vi "run_experiment_sCMOS_DAC_debug.vi"() -> ()   [LabVIEW 2015]
uses:
  <vilib>/addons/h5labview2/base/hid_t.ctl
  <vilib>/addons/h5labview2/base/H5Equery.vi
  <vilib>/addons/h5labview2/base/lib_path.vi
  <vilib>/DAQmx/write.llb/DAQmx Write (Digital Bool 1Line 1Point).vi
  <vilib>/addons/h5labview2/dataset/H5Dwrite.llb/H5Dwrite.xnode
  <vilib>/addons/h5labview2/dataset/H5D.lvlib
  <vilib>/addons/h5labview2/space/H5S.lvlib
  <vilib>/addons/h5labview2/file/H5F.lvlib
  <vilib>/DAQmx/read.llb/DAQmx Read (Analog 1D Wfm NChan NSamp).vi
  <vilib>/DAQmx/create/channels.llb/DAQmx Create Channel (DO-Digital Output).vi
  <vilib>/DAQmx/write.llb/DAQmx Write (Analog 1D DBL 1Chan NSamp).vi
panel:
  out "startrec err":errorcluster
  out "number of samples written per channel":u32
  out "error out 2":errorcluster
  out "temp .dcimg filepath":path
  out "Exposure":dbl
  out "V Width":i32
  out "H Width":i32
  out "Acquiring Frames":bool
  out "Frames Recorded":i32
  out "Display":T1(plugin-control)
  out "DAC Input":waveform(dbl)[](graph) caption="DAC Input Display"
  out "error out":errorcluster
  out "Current Stimulus Name":string
  out "Current Piezo Command":dynamicdata(graph)
  out "Current Stim Frames":i32
  out "Current Stim Duration":dbl
  out "Current Stimulus Save Path":path
  in  "Number Reps":dbl
  out "Experiment Path":path
  out "Timestamp":string
  out "Genotype":string
  out "Fly Name":string
  out "Experiment Name":string
  in  "Metadata Path":path
  out "Stimulus Files":path[](array[path])
  out "Num Stimuli":i32
  out "Protocol Name":string
  out "Protocol Rate":i32
  in  "Protocol Path":path
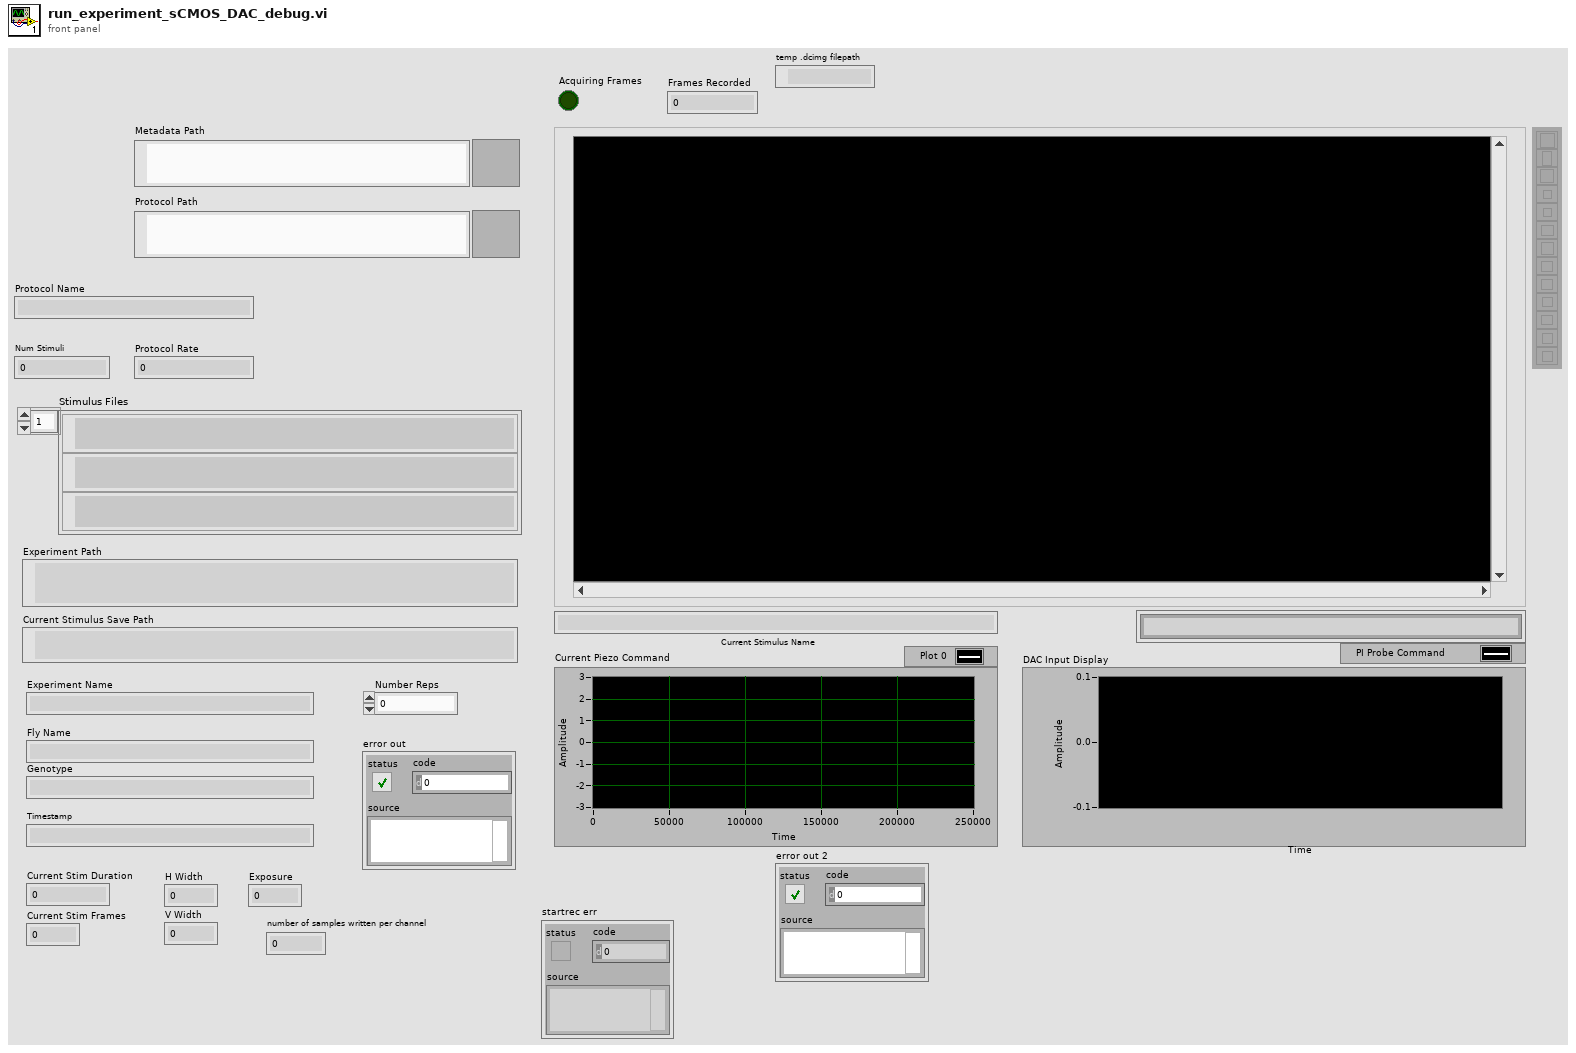
[diagram p1: front panel]
types:
  T1 = typedef "IMAQ Image.ctl" = refnum<image>
  T2 = cluster{"Value":i32, "Minimum":i32, "Maximum":i32, "Increment":i32}
  T3 = typedef "Image Type" = u32
  T4 = cluster{"height":u32, "width":u32, "datatype":u32}
  T5 = typedef "hid_t.ctl" = i32
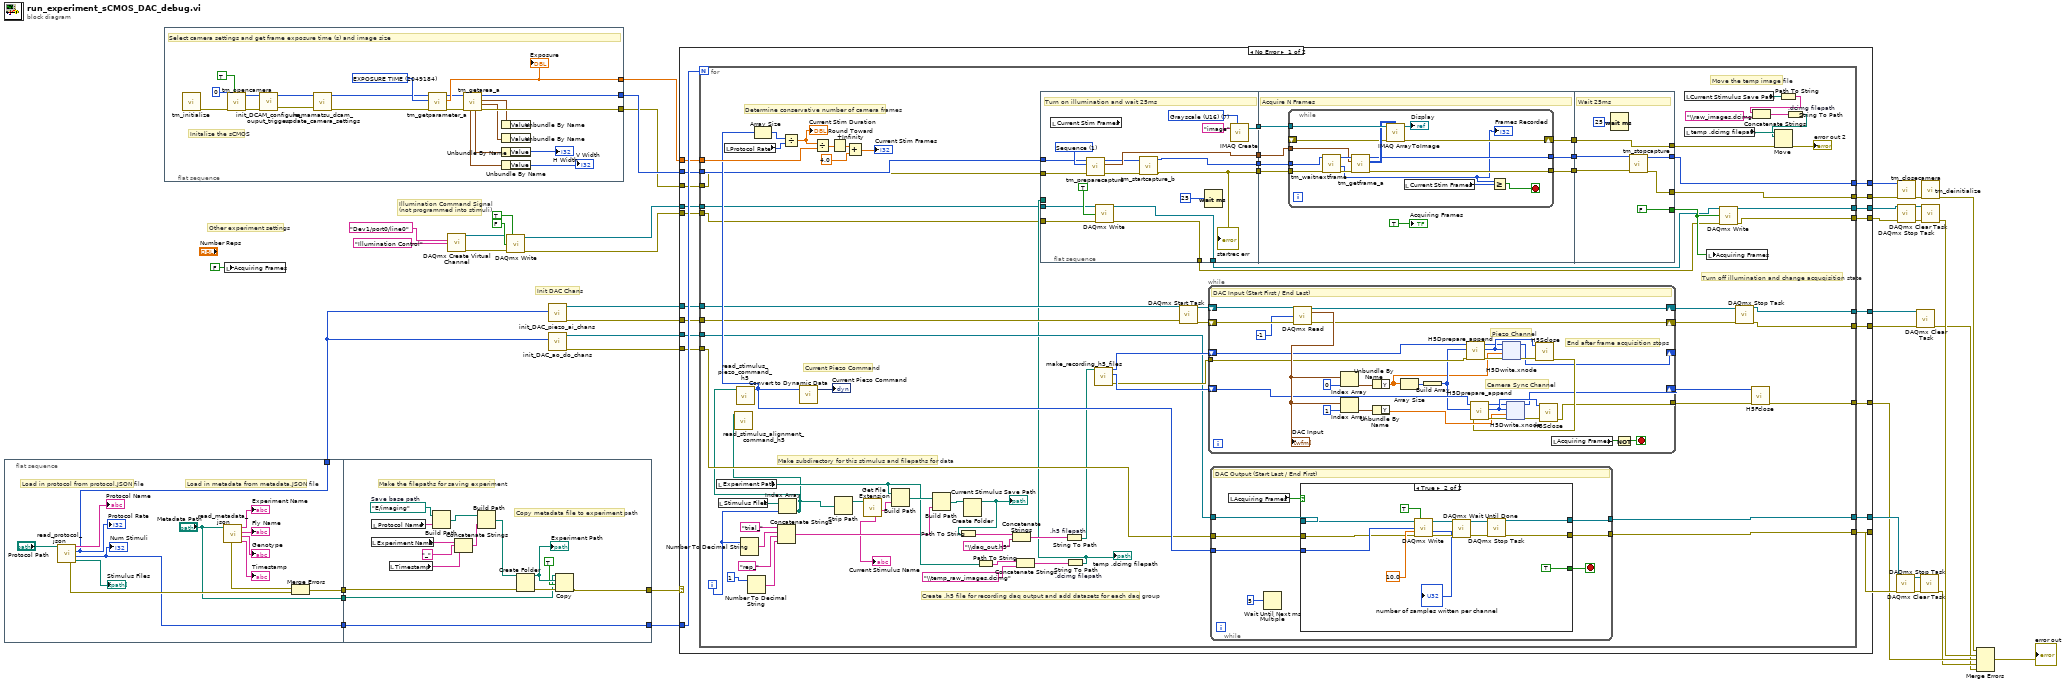
[diagram p0: block diagram]
diagram:
  # "Other experiment settings"
  # "Init DAC Chans"
  # "Illumination Command Signal \n(not programmed into stimuli)"
  n1 = flat-sequence {
    tunnel: [w44] -> w38
    tunnel: [w45] -> w10
    tunnel: ["Metadata Path"] -> w9
    tunnel: [w42] -> w8
    tunnel: [w69] -> w37
    tunnel: w10 -> [w57]
    tunnel: w9 -> [w56]
    tunnel: w8 -> [w69]
    tunnel: [w55] -> w7
    frame #0 {
      # "Load in metadata from metadata.JSON file"
      # "Load in protocol from protocol.JSON file"
      n2 = call "read_protocol_json.vi"("Path"="Protocol Path") -> ("stims"=→"Stimulus Files":path[], "n_stims"=w42:i32, "rate"=w44:i32, "protocol name"=→"Protocol Name":string, "error out"=w47:errorcluster)  [unwired: 6 in]
      "Protocol Rate" <- w44
      "Num Stimuli" <- w42
      n3 = call "read_metadata_json.vi"("Path"="Metadata Path") -> ("exp_time"=→"Timestamp":string, "genotype"=→"Genotype":string, "fly_name"=→"Fly Name":string, "exp_ name"=→"Experiment Name":string, "error out"=w46:errorcluster)  [unwired: 6 in]
      n4 = Merge Errors(w46, w47) -> (w45:errorcluster)
    }
    frame #1 {
      w64 = path "E:/imaging"  # Save base path
      # "Copy metadata file to experiment path"
      # "Make the filepaths for saving experiment"
      n5 = local read "Experiment Name"() -> (w61:string)
      n6 = local read "Protocol Name"() -> (w63:string)
      n7 = local read "Timestamp"() -> (w59:string)
      n8 = Build Path(base path=w64, name or relative path=w63) -> (appended path=w62:path)
      n9 = Concatenate Strings(w61, "_", w59) -> (w58:string)
      n10 = Build Path(base path=w62, name or relative path=w58) -> (appended path=w65:path)
      n11 = Create Folder(path (use dialog)=w65, error in=w57) -> (created path=w68:path, error out=w67:errorcluster)  [unwired: 1 in, 1 out]
      "Experiment Path" <- w68
      n12 = Copy(8:w67, 9:TRUE ("overwrite (F)"), 10:w68, 11:w56) -> (0:w55:errorcluster)  [unwired: 1 in, 2 out]
    }
  }
  n13 = flat-sequence {
    tunnel: [w89] -> w5
    tunnel: [w88] -> w4
    tunnel: [w90] -> w6
    frame #0 {
      w82 = u32 2049184 items=["SENSOR MODE"=4212128, "CCD MODE"=4212384, "READOUT MODE"=4211872, "ACTIVE VIEW INDEX"=4343136, "BITS PER CHANNEL"=4342976, "IMAGE PIXEL TYPE"=4343296, "BINNING"=4215968, "EXPOSURE TIME"=2049184, "CONTRAST GAIN"=3163312, "CONTRAST OFFSET"=3163328, "LIGHT MODE"=2114720, "SENSITIVITY"=2114992, "PHOTON IMAGING MODE"=2115200, "HIGH DYNAMIC RANGE MODE"=3163360, "WHITE BALANCE"=3163568, "TEMPERATURE"=2115232, "TEMPERATURE TARGET"=2115264, "SENSOR COOLER FAN"=2115296, "LINEBUNDLE HEIGHT"=4212192, "MECHANICAL SHUTTER"=2115488, "BACK FOCUS POSITION"=8422304, "TRIGGER CONNECTOR"=1066432, "TRIGGER SOURCE"=1066144, "OUTPUT TRIGGER SOURCE"=1852576, "TRIGGER GLOBAL EXPOSURE"=2049680, "FIRST TRIGGER BEHAVIOR"=2049696, "CHANNEL SYNC"=1852352, "READOUT DIRECTION"=4211904, "PRE HSYNC COUNT"=1852704] ("Parameter")
      # "Initalize the sCMOS"
      # "Select camera settings and get frame exposure time (s) and image size"
      n14 = call <userlib>:"tm_initialize.vi"() -> ("error out"=w87:errorcluster)  [unwired: 8 in, 3 out]
      n15 = call <userlib>:"tm_opencamera.vi"("Force Open"=TRUE, "error in (no error)"=w87, "Camera Index"=0) -> ("error out"=w83:errorcluster, "Handle out"=w84:u32)  [unwired: 6 in, 1 out]
      n16 = call "init_DCAM_configure_ouput_triggers.vi"("error in (no error)"=w83, "Handle in"=w84) -> ("error out"=w70:errorcluster, "Handle out"=w71:u32)  [unwired: 2 in]
      n17 = call "hamamatsu_dcam_update_camera_settings.vi"("error in (no error)"=w70, "Handle in"=w71) -> ("error out"=w73:errorcluster, "Handle out"=w72:u32)  [unwired: 6 in]
      n18 = call <userlib>:"tm_getparameter_a.vi"("error in (no error)"=w73, "Parameter"=w82, "Handle in"=w72) -> ("error out"=w77:errorcluster, "Value out"=w90:dbl, "Handle out"=w76:u32)  [unwired: 6 in]
      "Exposure" <- w90
      n19 = call <userlib>:"tm_getarea_a.vi"("error in (no error)"=w77, "Handle in"=w76) -> ("error out"=w88:errorcluster, "V Offset"=w80:T2, "H Offset"=w81:T2, "Handle out"=w89:u32, "H Width"=w79:T2, "V Width"=w78:T2)  [unwired: 4 in]
      n20 = Unbundle By Name(w81) -> ()  [unwired: 1 out]
      n21 = Unbundle By Name(w80) -> ()  [unwired: 1 out]
      n22 = Unbundle By Name(w79) -> ("Value"=→"H Width":i32)
      n23 = Unbundle By Name(w78) -> ("Value"=→"V Width":i32)
    }
  }
  n24 = local write "Acquiring Frames"(FALSE ("Acquiring Frames")) -> ()
  n25 = call-poly <vilib>:"DAQmx Create Virtual Channel.vi"("lines"=tag "Dev1/port0/line0" ("DAQmx Physical Channel"), "name to assign"="Illumination Control") -> ("task out"=w2:refnum<k21>, "error out"=w1:errorcluster)  [unwired: 12 in]
  n26 = call-poly <vilib>:"DAQmx Write.vi"("task/channels in"=w2, "auto start"=TRUE, "data"=FALSE, "error in"=w1) -> ("task out"=w16:refnum<k21>, "error out"=w15:errorcluster)  [unwired: 9 in, 1 out]
  n27 = call "init_DAC_piezo_ai_chans.vi"("Sample Rate"=w38) -> ("error out"=w13:errorcluster, "Refnum out"=w14:refnum<k21>)  [unwired: 8 in, 1 out]
  n28 = call "init_DAC_ao_do_chans.vi"("Rate"=w38) -> ("error out"=w11:errorcluster, "AO Out"=w12:refnum<k21>)  [unwired: 8 in, 1 out]
  n29 = case shown="No Error" w7 {
    tunnel: w37 -> [w109 _]
    tunnel: w6 -> [w108 _]
    tunnel: w5 -> [w107 w326]
    tunnel: w4 -> [w106 w325]
    tunnel: [w100 _] -> w24
    tunnel: [w99 _] -> w25
    tunnel: [w105 _] -> w28
    tunnel: [w104 _] -> w29
    tunnel: [w103 w325] -> w21
    tunnel: [w102 w326] -> w20
    tunnel: [w101 _] -> w27
    tunnel: [w98 _] -> w19
    tunnel: [w97 _] -> w18
    tunnel: w16 -> [w96 _]
    tunnel: w15 -> [w95 _]
    tunnel: w14 -> [w94 _]
    tunnel: w13 -> [w93 _]
    tunnel: w12 -> [w92 _]
    tunnel: w11 -> [w91 _]
    frame No Error {
      n30 = for {
        N: w109 -> [_]
        tunnel: w108 -> [w180]
        tunnel: w107 -> [w146]
        tunnel: w106 -> [w145]
        tunnel: [w172] -> w105
        tunnel: [w171] -> w104
        tunnel: [w124] -> w103
        tunnel: [w125] -> w102
        tunnel: [w166] -> w101
        tunnel: [w162] -> w100
        tunnel: [w161] -> w99
        tunnel: [w160] -> w98
        tunnel: [w159] -> w97
        tunnel: w96 -> [w128]
        tunnel: w95 -> [w129]
        tunnel: w94 -> [w158]
        tunnel: w93 -> [w157]
        tunnel: w92 -> [w156]
        tunnel: w91 -> [w155]
        i -> [w184]
        # "Move the temp image file"
        # "Create .h5 file for recording daq output and add datasets for each daq group"
        # "Current Piezo Command"
        # "Turn off illumination and change acquqisition state"
        # "Determine conservative number of camera frames"
        # "Make subdirectory for this stimulus and filepaths for data"
        n31 = local read "Experiment Path"() -> (w134:path)
        n32 = local read "Stimulus Files"() -> (w185:path[])
        n33 = local read "Protocol Rate"() -> (w111:i32)
        n34 = Number To Decimal String(number=w184) -> (decimal integer string=w187:string)  [unwired: 1 in]
        n35 = Number To Decimal String(number=i16 1 ("width (-)")) -> (decimal integer string=w182:string)  [unwired: 1 in]
        n36 = Concatenate Strings("trial_", w187, "rep_", w182) -> (w132:string)
        n37 = Index Array(array=w185, index=w184) -> (element=w133:path)
        n38 = call "read_stimulus_alignment_command_h5.vi"("Path"=w133) -> ()  [unwired: 9 in, 2 out]
        n39 = call "read_stimulus_piezo_command_h5.vi"("Path"=w133) -> ("stimulus"=w165:i32[])  [unwired: 9 in, 1 out]
        n40 = Array Size(array=w165) -> (size(s)=w112:i32)
        n41 = Divide(x=w112, y=w111) -> (x/y=w110:dbl)
        "Current Stim Duration" <- w110
        n42 = call "Convert to Dynamic Data"("Array"=w165) -> ("Dynamic Data Type"=→"Current Piezo Command":dynamicdata)  [unwired: 3 in]
        n43 = Divide(x=w110, y=w180) -> (x/y=w179:dbl)
        n44 = Round Toward +Infinity(x=w179) -> (ceil(x): smallest int >= x=w178:dbl)
        n45 = Strip Path(path=w133) -> (stripped path=w138:path)  [unwired: 1 out]
        n46 = Add(x=w178, y=4.0) -> (x+y=→"Current Stim Frames":dbl)
        n47 = call <vilib>:"Get File Extension.vi"("file"=w138) -> ("filename without extension"=w139:string, "unmodified file extension"=→"Current Stimulus Name":string)  [unwired: 6 in, 3 out]
        n48 = Build Path(base path=w134, name or relative path=w139) -> (appended path=w140:path)
        n49 = Build Path(base path=w140, name or relative path=w132) -> (appended path=w141:path)
        n50 = Create Folder(path (use dialog)=w141) -> (created path=w123:path)  [unwired: 2 in, 2 out]
        "Current Stimulus Save Path" <- w123
        n51 = Path To String(path=w123) -> (string=w136:string)
        n52 = Path To String(path=w134) -> (string=w142:string)
        n53 = Concatenate Strings(w136, "\\daq_out.h5" ("string")) -> (w135:string)
        n54 = Concatenate Strings(w142, "\\temp_raw_images.dcimg" ("string")) -> (w144:string)
        n55 = flat-sequence {
          tunnel: [w188] -> w154
          tunnel: [w200] -> w153
          tunnel: [w189] -> w152
          tunnel: [w197] -> w151
          tunnel: w146 -> [w202]
          tunnel: w145 -> [w201]
          tunnel: w130 -> [_]
          tunnel: w129 -> [w195]
          tunnel: w128 -> [w194]
          tunnel: [w193] -> w127
          tunnel: [w192] -> w126
          tunnel: w154 -> [w211]
          tunnel: w153 -> [w210]
          tunnel: w152 -> [w209]
          tunnel: [w208] -> w150
          tunnel: [w207] -> w149
          tunnel: w151 -> [w206]
          tunnel: [w205] -> w148
          tunnel: [FALSE] -> w147
          tunnel: w150 -> [w228]
          tunnel: w149 -> [w229]
          tunnel: [w230] -> w124
          tunnel: [w231] -> w125
          tunnel: w148 -> [w232]
          tunnel: [w232] -> w113
          frame #0 {
            w199 = T3 7 items=["Grayscale (U8)", "Grayscale (I16)", "Grayscale (SGL)", "Complex (CSG)", "RGB (U32)", "HSL (U32)", "RGB (U64)", "Grayscale (U16)"] ("Image Type")
            w203 = 1 items=["Snap", "Sequence"] ("Capture mode")
            # "Turn on illumination and wait 25ms"
            n56 = local read "Current Stim Frames"() -> ()  [unwired: 1 out]
            n57 = call <userlib>:"tm_preparecapture.vi"("error in (no error)"=w201, "Capture mode"=w203, "Handle in"=w202) -> ("error out"=w191:errorcluster, "Buffer Info"=w200:T4, "Handle out"=w190:u32)  [unwired: 5 in, 1 out]
            n58 = call-poly <vilib>:"DAQmx Write.vi"("task/channels in"=w194, "data"=TRUE, "error in"=w195) -> ("task out"=w193:refnum<k21>, "error out"=w192:errorcluster)  [unwired: 10 in, 1 out]
            n59 = call <userlib>:"tm_startcapture_b.vi"("error in (no error)"=w191, "Handle in"=w190) -> ("error out"=w188:errorcluster, "Handle out"=w189:u32)  [unwired: 8 in]
            "startrec err" <- w188
            n60 = Wait (ms)(milliseconds to wait=u32 25) -> ()  [unwired: 1 out]
            n61 = call "IMAQ Create"("Image Name"="image", "Image Type"=w199) -> ("New Image"=w197:T1)  [unwired: 3 in, 1 out]
          }
          frame #1 {
            # "Acquire N Frames"
            n62 = while {
              tunnel: w211 -> [w225]
              tunnel: w210 -> [w224]
              tunnel: w209 -> [w223]
              tunnel: [w214] -> w208
              tunnel: [w215] -> w207
              tunnel: w206 -> [w220]
              shift-right: [w218] -> w205
              shift-left: _ -> [w217]
              stop <- w221 stop-if-true
              n63 = call <userlib>:"tm_waitnextframe.vi"("error in (no error)"=w225, "Handle in"=w223) -> ("error out"=w227:errorcluster, "Frame Count"=w213:i32, "Handle out"=w226:u32)  [unwired: 6 in, 1 out]
              "Frames Recorded" <- w213
              n64 = call <userlib>:"tm_getframe_a.vi"("error in (no error)"=w227, "Buffer Info"=w224, "Handle in"=w226) -> ("error out"=w215:errorcluster, "Data 16"=w219:u16[][], "Handle out"=w214:u32)  [unwired: 4 in, 2 out]
              n65 = call "IMAQ ArrayToImage"("Image Pixels (U16)"=w219, "error in (no error)"=w217, "Image"=w220) -> ("error out"=w218:errorcluster, "Image Out"=→"Display":T1)  [unwired: 7 in]
              n66 = local read "Current Stim Frames"() -> (w222:i32)
              n67 = Greater Or Equal?(x=w213, y=w222) -> (x >= y?=w221:bool)
            }
            "Acquiring Frames" <- TRUE
          }
          frame #2 {
            # "Wait 25ms"
            n68 = Wait (ms)(milliseconds to wait=u32 25) -> ()  [unwired: 1 out]
            n69 = call <userlib>:"tm_stopcapture.vi"("error in (no error)"=w229, "Handle in"=w228) -> ("error out"=w230:errorcluster, "Handle out"=w231:u32)  [unwired: 8 in]
          }
        }
        n70 = String To Path ".h5 filepath"(string=w135) -> (path=w131:path)
        n71 = String To Path ".dcimg filepath"(string=w144) -> (path=w130:path)
        "temp .dcimg filepath" <- w130
        n72 = call "make_recording_h5_files.vi"("Path"=w131) -> ("error out"=w175:errorcluster, "Camera Dataset"=w176:T5, "Piezo Dataset"=w174:T5)  [unwired: 8 in]
        n73 = call <vilib>:"DAQmx Start Task.vi"("task/channels in"=w158, "error in"=w157) -> ("task out"=w170:refnum<k21>, "error out"=w169:errorcluster)  [unwired: 12 in]
        n74 = while {
          tunnel: w175 -> [w274]
          shift-right: [w263] -> w168
          shift-left: w176 -> [w269]
          shift-right: [w264] -> _
          shift-left: w174 -> [w275]
          tunnel: [w262] -> w167
          shift-right: [w260] -> w164
          shift-left: w170 -> [w288]
          shift-right: [w259] -> w163
          shift-left: w169 -> [w287]
          stop <- w261 stop-if-true
          # "End after frame acquisition stops"
          # "Camera Sync Channel"
          # "Piezo Channel"
          # "DAC Input (Start First / End Last)"
          n75 = call-poly <vilib>:"DAQmx Read.vi"("task/channels in"=w288, "number of samples per channel"=-1, "error in"=w287) -> ("task out"=w260:refnum<k21>, "data"=w281:waveform(dbl)[], "error out"=w259:errorcluster)  [unwired: 10 in]
          "DAC Input" <- w281
          n76 = Index Array(array=w281, index=0) -> (element=w285:waveform(dbl))
          n77 = Index Array(array=w281, index=1) -> (element=w283:waveform(dbl))
          n78 = Unbundle By Name(w285) -> ("Y"=w266:dbl[])
          n79 = Unbundle By Name(w283) -> ("Y"=w267:dbl[])
          n80 = Array Size(array=w266) -> (size(s)=w276:i32)
          n81 = Build Array(w276) -> (w268:i32[])
          n82 = call <vilib>:"H5Dprepare_append.vi"("error in (no error)"=w274, "append dims"=w268, "dset in"=w275) -> ("error out"=w277:errorcluster, "space out"=w280:T5, "dset out"=w278:T5)  [unwired: 6 in]
          n83 = xnode "H5Dwrite.xnode"("error in (no error)"=w277, "data"=w266, "file space"=w280, "ref in"=w278) -> ("error out"=w279:errorcluster, "ref out"=w264:T5)  [unwired: 3 in, 1 out]
          n84 = call <vilib>:"H5Sclose.vi"("error in (no error)"=w279, "space in"=w280) -> ("error out"=w265:errorcluster)  [unwired: 9 in]
          n85 = call <vilib>:"H5Dprepare_append.vi"("error in (no error)"=w265, "append dims"=w268, "dset in"=w269) -> ("error out"=w270:errorcluster, "space out"=w273:T5, "dset out"=w271:T5)  [unwired: 6 in]
          n86 = xnode "H5Dwrite.xnode"("error in (no error)"=w270, "data"=w267, "file space"=w273, "ref in"=w271) -> ("error out"=w272:errorcluster, "ref out"=w263:T5)  [unwired: 3 in, 1 out]
          n87 = call <vilib>:"H5Sclose.vi"("error in (no error)"=w272, "space in"=w273) -> ("error out"=w262:errorcluster)  [unwired: 9 in]
          n88 = local read "Acquiring Frames"() -> (w258:bool)
          n89 = Not(x=w258) -> (.not. x?=w261:bool)
        }
        n90 = while {
          tunnel: w165 -> [w240]
          tunnel: w156 -> [w236]
          tunnel: [w238] -> w171
          tunnel: [w237] -> w172
          tunnel: w155 -> [w235]
          stop <- w241 stop-if-true
          # "DAC Output (Start Last / End First)"
          n91 = local read "Acquiring Frames"() -> (w242:bool)
          n92 = Wait Until Next ms Multiple(millisecond multiple=u32 5) -> ()  [unwired: 1 out]
          n93 = case shown="True" w242 {
            tunnel: [_ TRUE] -> w241
            tunnel: w235 -> [w243 w250]
            tunnel: w236 -> [w244 w251]
            tunnel: w240 -> [_ w253]
            tunnel: [w244 w255] -> w238
            tunnel: [w243 w254] -> w237
            frame False {
            }
            frame True {
              n94 = call-poly <vilib>:"DAQmx Write.vi"("task/channels in"=w251, "auto start"=TRUE, "data"=w253, "timeout"=10.0, "error in"=w250) -> ("task out"=w247:refnum<k21>, "number of samples written per channel"=→"number of samples written per channel":u32, "error out"=w246:errorcluster)  [unwired: 8 in]
              n95 = call <vilib>:"DAQmx Wait Until Done.vi"("task/channels in"=w247, "error in"=w246) -> ("task out"=w249:refnum<k21>, "error out"=w248:errorcluster)  [unwired: 12 in]
              n96 = call <vilib>:"DAQmx Stop Task.vi"("task/channels in"=w249, "error in"=w248) -> ("task out"=w255:refnum<k21>, "error out"=w254:errorcluster)  [unwired: 12 in]
            }
          }
        }
        n97 = local read "Current Stimulus Save Path"() -> (w115:path)
        n98 = local read "temp .dcimg filepath"() -> (w119:path)
        n99 = local write "Acquiring Frames"(w147) -> ()
        n100 = call-poly <vilib>:"DAQmx Write.vi"("task/channels in"=w127, "data"=w147, "error in"=w126) -> ("task out"=w162:refnum<k21>, "error out"=w161:errorcluster)  [unwired: 10 in, 1 out]
        n101 = call <vilib>:"DAQmx Stop Task.vi"("task/channels in"=w164, "error in"=w163) -> ("task out"=w159:refnum<k21>, "error out"=w160:errorcluster)  [unwired: 12 in]
        n102 = call <vilib>:"H5Fclose.vi"("error in (no error)"=w167, "ref"=w168) -> ("error out"=w166:errorcluster)  [unwired: 9 in]
        n103 = Path To String(path=w115) -> (string=w116:string)
        n104 = Concatenate Strings(w116, "\\raw_images.dcimg" ("string")) -> (w118:string)
        n105 = String To Path ".dcimg filepath"(string=w118) -> (path=w114:path)
        n106 = Move(source path=w119, error in=w113, 10:w114) -> (error out=→"error out 2":errorcluster)  [unwired: 2 in, 2 out]
      }
    }
    frame Error {
    }
  }
  n107 = call <vilib>:"DAQmx Stop Task.vi"("task/channels in"=w29, "error in"=w28) -> ("task out"=w31:refnum<k21>, "error out"=w30:errorcluster)  [unwired: 12 in]
  n108 = call <userlib>:"tm_closecamera.vi"("error in (no error)"=w21, "Handle in"=w20) -> ("error out"=w32:errorcluster)  [unwired: 9 in]
  n109 = call <vilib>:"DAQmx Stop Task.vi"("task/channels in"=w24, "error in"=w25) -> ("task out"=w34:refnum<k21>, "error out"=w33:errorcluster)  [unwired: 12 in]
  n110 = call <vilib>:"DAQmx Clear Task.vi"("task in"=w18, "error in"=w19) -> ("error out"=w17:errorcluster)  [unwired: 13 in]
  n111 = call <vilib>:"DAQmx Clear Task.vi"("task in"=w31, "error in"=w30) -> ("error out"=w26:errorcluster)  [unwired: 13 in]
  n112 = call <userlib>:"tm_deinitialize.vi"("error in (no error)"=w32) -> ("error out"=w22:errorcluster)  [unwired: 10 in]
  n113 = call <vilib>:"DAQmx Clear Task.vi"("task in"=w34, "error in"=w33) -> ("error out"=w23:errorcluster)  [unwired: 13 in]
  n114 = Merge Errors(w22, w23, w27, w26, w17) -> (→"error out":errorcluster)
